vi "SaveNumericArrayToTDMS.vi"(0 "tdms file ref in":refnum<k34>, 5 "Array of Channels":string[](array[string]), 7 "Group Name":string, 9 "Array of Values":dbl[](array[numeric]), 11 "error in (no error)":errorcluster) -> (4 "tdms file ref out":refnum<k34>, 15 "error out":errorcluster)   [LabVIEW 2014]
uses:
  Variables/Physical data.vi
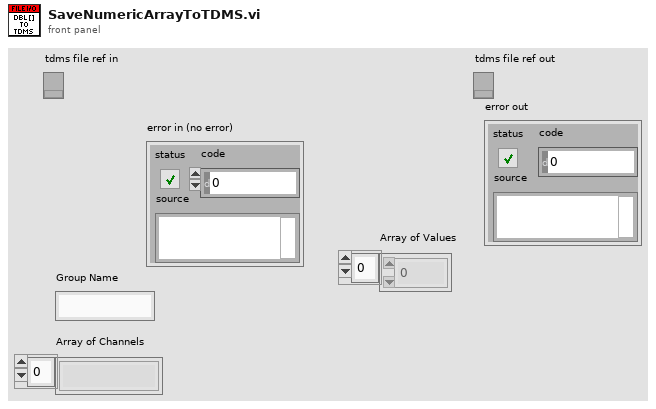
[diagram p1: front panel]
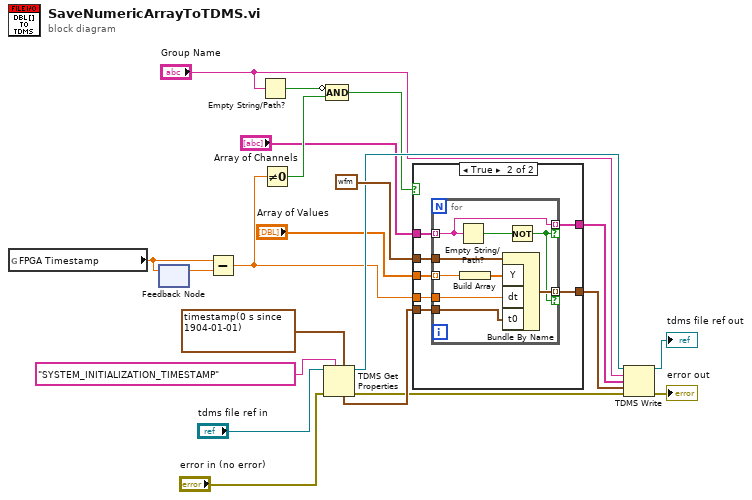
[diagram p0: block diagram]
diagram:
  n1 = global read "Physical data.vi" "FPGA Timestamp"() -> (w10:dbl)
  n2 = feedback-in #1(w10) -> ()
  n3 = feedback #1() -> (w16:dbl)  [unwired: 1 in]
  n4 = Subtract(x=w10, y=w16) -> (x-y=w9:dbl)
  n5 = Empty String/Path?(string/path="Group Name") -> (empty?=w6:bool)
  n6 = Not Equal To 0?(x=w9) -> (x != 0?=w7:bool)
  n7 = TDMS Get Properties(5:timestamp(0 s since 1904-01-01) ("current time"), 7:"SYSTEM_INITIALIZATION_TIMESTAMP", 8:"error in (no error)", 11:"tdms file ref in") -> (0:w12:errorcluster, 3:w13:refnum<k34>, 4:w17:timestamp)  [unwired: 2 in, 3 out]
  n8 = Compound Arithmetic op=AND(invert w6, w7) -> (w5:bool)
  n9 = case shown="True" w5 {
    tunnel: w17 -> [_ w28]
    tunnel: waveform(dbl) {"t0"=timestamp(0 s since 1904-01-01), "dt"=1.0, "Y"=[]} ("Waveform") -> [_ w27]
    tunnel: [_ w26] -> w14
    tunnel: "Array of Values" -> [_ w25]
    tunnel: w9 -> [_ w24]
    tunnel: "Array of Channels" -> [_ w23]
    tunnel: [_ w22] -> w3
    frame False {
    }
    frame True {
      n10 = for {
        tunnel: w28 -> [w36]
        tunnel: w27 -> [w37]
        tunnel: w24 -> [w35]
        tunnel: [w34] -> w26 mode=indexing if=w29
        tunnel: w25 -> [w33] mode=indexing
        tunnel: w23 -> [w30] mode=indexing
        tunnel: [w30] -> w22 mode=indexing if=w29
        n11 = Empty String/Path?(string/path=w30) -> (empty?=w31:bool)
        n12 = Build Array(w33) -> (w32:dbl[])
        n13 = Bundle By Name(cluster=w37, "Y"=w32, "dt"=w35, "t0"=w36) -> (w34:waveform(dbl))
        n14 = Not(x=w31) -> (.not. x?=w29:bool)
      }
    }
  }
  n15 = TDMS Write(0:w13, 5:"Group Name", 7:w3, 9:w14, 11:w12) -> (4:→"tdms file ref out":refnum<k34>, 15:→"error out":errorcluster)  [unwired: 1 in, 2 out]
